vi "testInsert.vi"(8 "error in (no error)":errorcluster, 11 "TestCase in":refnum<class "StringList_Delegations.lvclass">) -> (0 "error out":errorcluster, 3 "TestCase out":refnum<class "StringList_Delegations.lvclass">)   [LabVIEW 2013, in "StringList_Delegations.lvclass"]
uses:
  StringList_Delegations.lvclass
  StringList_Delegations.lvclass/StringList_Delegations.ctl
  source/LapDog.Collections.Lists/StringList/StringList.lvclass
  <vilib>/addons/_JKI Toolkits/VI Tester/TestCase.llb/TestCase.lvclass
  UnitTestComparisons/UnitTestComparisons.lvlib
  Test Doubles/ListImp_RefSpy/ListImp_RefSpy.lvclass
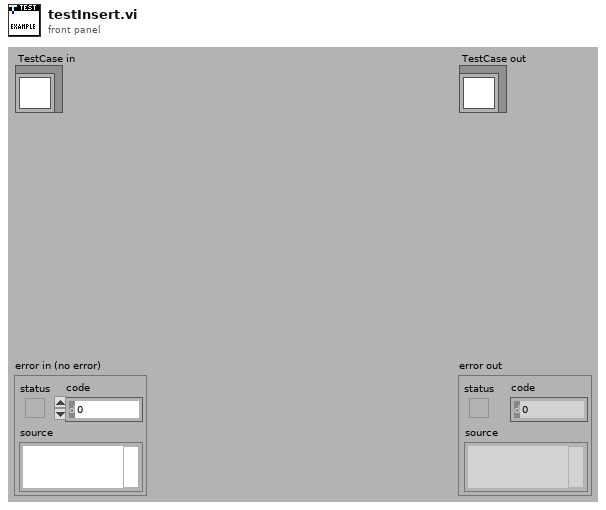
[diagram p1: front panel]
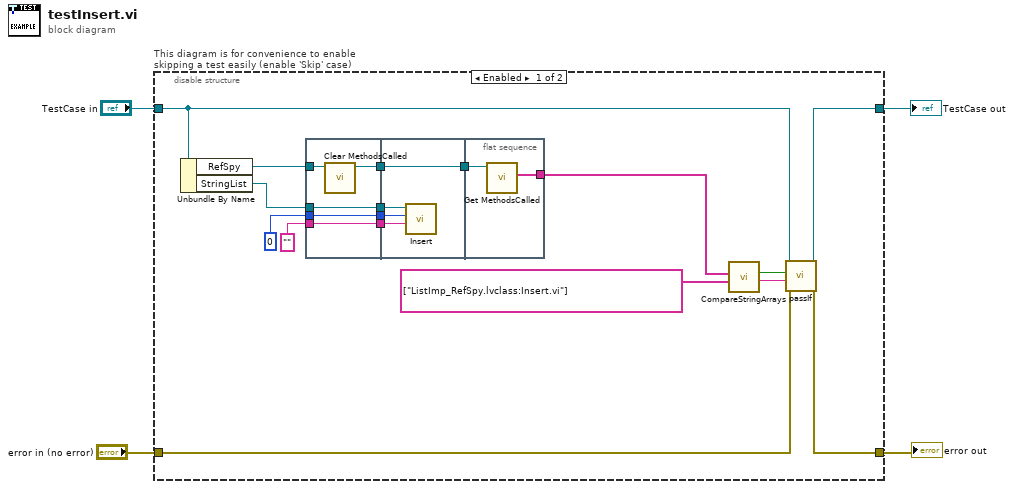
[diagram p0: block diagram]
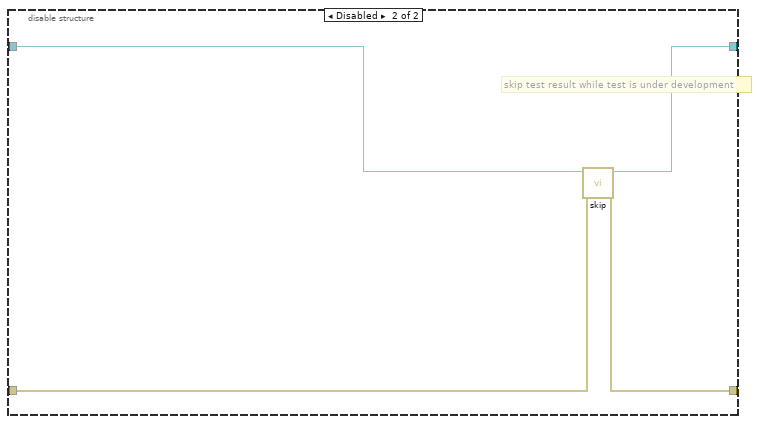
[diagram p2: hidden frame]
diagram:
  n1 = disable-structure "This diagram is for convenience to enable skipping a test easily (enable 'Skip' case)" shown="Enabled" {
    disable-tunnel: "TestCase in" -> [w16 w36]
    disable-tunnel: [w21 w34] -> w1
    disable-tunnel: [w20 w35] -> w3
    disable-tunnel: "error in (no error)" -> [w19 w33]
    frame Enabled {
      n2 = Unbundle By Name(w16) -> ("RefSpy"=w13:refnum<class "ListImp_RefSpy.lvclass">, "StringList"=w15:refnum<class "StringList.lvclass">)
      n3 = flat-sequence {
        tunnel: w13 -> [w25]
        tunnel: w15 -> [w26]
        tunnel: [w26] -> w10
        tunnel: [w24] -> w9
        tunnel: 0 -> [w23]
        tunnel: [w23] -> w7
        tunnel: "" -> [w22]
        tunnel: [w22] -> w5
        tunnel: [w30] -> w14
        tunnel: w10 -> [w29]
        tunnel: w9 -> [w30]
        tunnel: w7 -> [w28]
        tunnel: w5 -> [w27]
        tunnel: w14 -> [w32]
        tunnel: [w31] -> w11
        frame #0 {
          n4 = call "Clear MethodsCalled.vi"("MockListImp in"=w25) -> ("MockListImp out"=w24:refnum<class "ListImp_RefSpy.lvclass">)  [unwired: 9 in, 1 out]
        }
        frame #1 {
          n5 = call-dynamic "Insert.vi"("String"=w27, "Index"=w28, "StringList in"=w29) -> ()  [unwired: 7 in, 2 out]
        }
        frame #2 {
          n6 = call "Get MethodsCalled.vi"("MockListImp"=w32) -> ("MethodsCalled"=w31:string[])  [unwired: 9 in, 1 out]
        }
      }
      n7 = call "CompareStringArrays.vi"("Expected Strings"=string[] ["ListImp_RefSpy.lvclass:Insert.vi"] ("Actual Strings"), "Actual Strings"=w11) -> ("Message"=w17:string, "Equal?"=w18:bool)  [unwired: 8 in]
      n8 = call-dynamic "passIf.vi"("error in (no error)"=w19, "message (\"\")"=w17, "pass"=w18, "TestCase in"=w16) -> ("error out"=w20:errorcluster, "TestCase out"=w21:refnum<class "StringList_Delegations.lvclass">)  [unwired: 6 in]
    }
    frame Disabled {
      # "skip test result while test is under development"
      n9 = call <vilib>:"skip.vi"("error in (no error)"=w33, "TestCase in"=w36) -> ("error out"=w35:errorcluster, "TestCase out"=w34:refnum<class "StringList_Delegations.lvclass">)  [unwired: 8 in]
    }
  }
  "error out" <- w3
  "TestCase out" <- w1
